vi "Stitch Together Images.vi"(8 "error in":errorcluster, 9 "Quality":enum16{"perfect", "medium", "low"}(ring), 10 "Physical Images in":T1[](array[typedef]), 11 "Image Dst":T2) -> (0 "error out":errorcluster, 2 "Physical Images out":T1[](array[typedef]), 3 "Composite Physical Image":T1)   [LabVIEW 2011]
uses:
  Type Definitions/Physical Image.ctl
  Vec3d Class/Vec3d Class.lvclass
  <vilib>/vision/Image Controls.llb/IMAQ Image.ctl
  <vilib>/vision/NI_Vision_Development_Module.lvlib
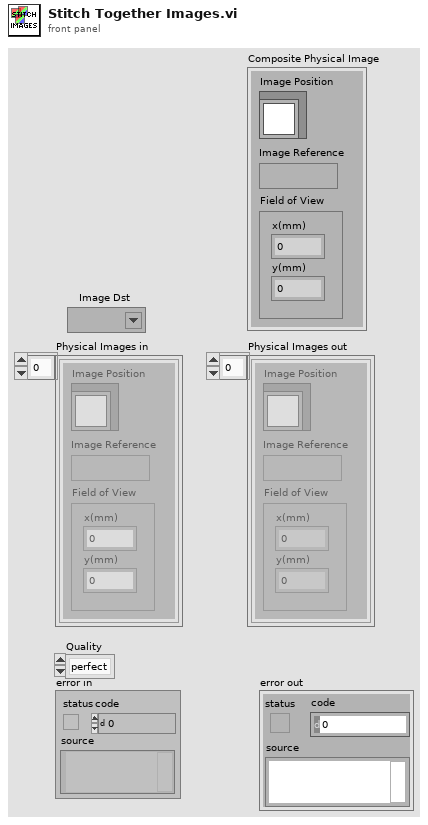
[diagram p1: front panel]
types:
  T1 = typedef "Physical Image.ctl" = cluster{"Image Position":refnum<class "Vec3d Class.lvclass">, "Image Reference":T2, "Field of View":cluster{"x(mm)":dbl, "y(mm)":dbl}}
  T2 = typedef "IMAQ Image.ctl" = refnum<image>
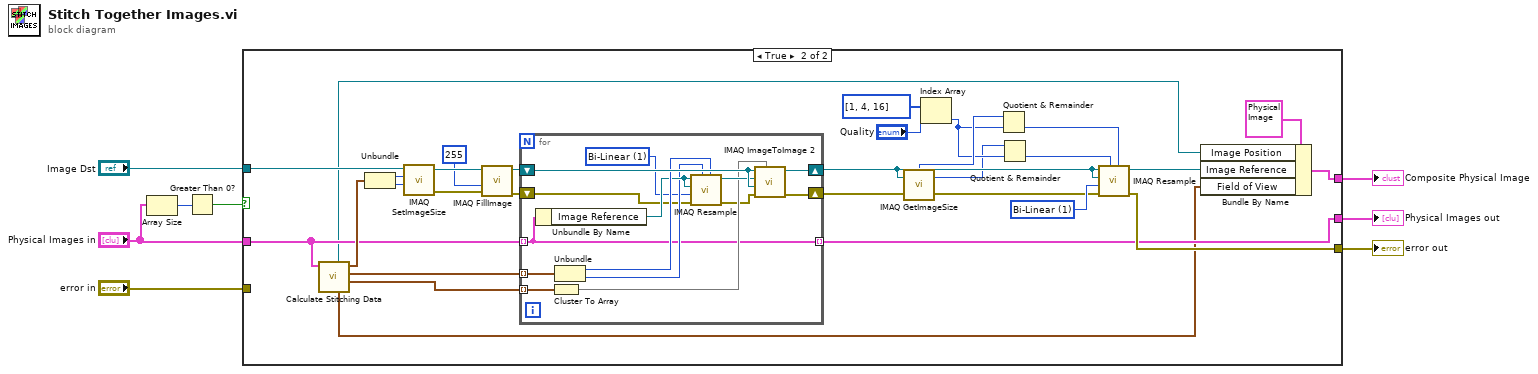
[diagram p0: block diagram]
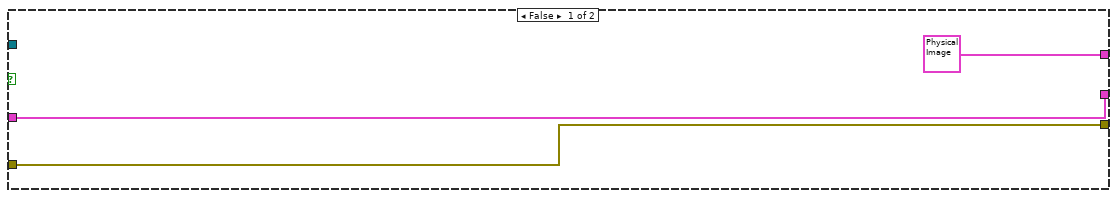
[diagram p2: hidden frame]
diagram:
  n1 = Array Size(array="Physical Images in") -> (size(s)=w7:i32)
  n2 = Greater Than 0?(x=w7) -> (x > 0?=w6:bool)
  n3 = case shown="True" w6 {
    tunnel: "Physical Images in" -> [w10 w17]
    tunnel: "Image Dst" -> [_ w41]
    tunnel: "error in" -> [w11 _]
    tunnel: [w11 w32] -> w4
    tunnel: [w10 w14] -> w3
    tunnel: [T1 {"Image Position"=refnum, "Image Reference"=refnum, "Field of View"={"x(mm)"=0.0, "y(mm)"=0.0}} ("Physical Image") w34] -> w1
    frame False {
    }
    frame True {
      w33 = u32 1 items=["Zero Order", "Bi-Linear", "Quadratic", "Cubic Spline"] ("Interpolation Type")
      n4 = call "Calculate Stitching Data.vi"("Physical Images in"=w17) -> ("Image overlay positions"=w15:cluster{i32, i32}[], "Image Rescale Resolutions"=w16:cluster{"Cols":i32, "Rows":i32}[], "Target Resolution"=w20:cluster{"cols":i32, "rows":i32}, "Target FOV"=w12:cluster{"x(mm)":dbl, "y(mm)":dbl}, "Target Center"=w13:refnum<class "Vec3d Class.lvclass">)  [unwired: 5 in, 1 out]
      n5 = Unbundle(w20) -> ("cols"=w19:i32, "rows"=w18:i32)
      n6 = call "IMAQ SetImageSize"("Y Resolution"=w18, "X Resolution"=w19, "Image"=w41) -> ("error out"=w37:errorcluster, "Image Out"=w40:T2)  [unwired: 2 in]
      n7 = call "IMAQ FillImage"("error in (no error)"=w37, "Pixel Value (U8, U16, I16, Float)"=u8 255, "Image"=w40) -> ("error out"=w36:errorcluster, "Image Out"=w39:T2)  [unwired: 7 in]
      n8 = for {
        shift-right: [w55] -> w28
        shift-left: w39 -> [w54]
        shift-right: [w53] -> w27
        shift-left: w36 -> [w46]
        tunnel: w17 -> [w42] mode=indexing
        tunnel: w16 -> [w52] mode=indexing
        tunnel: w15 -> [w45] mode=indexing
        tunnel: [w42] -> w14 mode=indexing
        w47 = u32 1 items=["Zero Order", "Bi-Linear", "Quadratic", "Cubic Spline"] ("Interpolation Type")
        n9 = Unbundle By Name(w42) -> ("Image Reference"=w49:T2)
        n10 = Cluster To Array(cluster=w45) -> (array=w44:i32[])
        n11 = Unbundle(w52) -> ("Cols"=w51:i32, "Rows"=w48:i32)
        n12 = call "IMAQ Resample"("X Resolution"=w51, "Y Resolution"=w48, "error in (no error)"=w46, "Interpolation Type"=w47, "Image Dst"=w49, "Image Src"=w49) -> ("error out"=w43:errorcluster, "Image Dst Out"=w50:T2)  [unwired: 4 in]
        n13 = call "IMAQ ImageToImage 2"("Offset Left/Top"=w44, "error in (no error)"=w43, "Image Dst"=w54, "Image Src (Small)"=w50, "Image Src (Large)"=w54) -> ("error out"=w53:errorcluster, "Image Dst Out"=w55:T2)  [unwired: 5 in]
      }
      n14 = call "IMAQ GetImageSize"("Image"=w28, "error in (no error)"=w27) -> ("Y Resolution"=w23:i32, "X Resolution"=w25:i32, "error out"=w26:errorcluster)  [unwired: 2 in]
      n15 = Index Array(array=i32[] [1, 4, 16], index="Quality") -> (element=w24:i32)
      n16 = Quotient & Remainder(x=w25, y=w24) -> (floor(x/y)=w22:i32)  [unwired: 1 out]
      n17 = Quotient & Remainder(x=w23, y=w24) -> (floor(x/y)=w21:i32)  [unwired: 1 out]
      n18 = call "IMAQ Resample"("X Resolution"=w22, "Y Resolution"=w21, "error in (no error)"=w26, "Interpolation Type"=w33, "Image Dst"=w28, "Image Src"=w28) -> ("error out"=w32:errorcluster, "Image Dst Out"=w31:T2)  [unwired: 4 in]
      n19 = Bundle By Name(cluster=T1 {"Image Position"=refnum, "Image Reference"=refnum, "Field of View"={"x(mm)"=0.0, "y(mm)"=0.0}} ("Physical Image"), "Image Position"=w13, "Image Reference"=w31, "Field of View"=w12) -> (w34:T1)
    }
  }
  "error out" <- w4
  "Physical Images out" <- w3
  "Composite Physical Image" <- w1
